vi "Send Set Room Lamp State.vi"(7 "Priority":T2=enum."Normal" caption="Message Priority (Normal)", 8 "error in (no error)":errorcluster, 9 "Value":bool, 10 "Room List":T1, 11 "Message Enqueuer in":refnum<class "Message Enqueuer.lvclass">) -> (0 "error out":errorcluster, 3 "Message Enqueuer out":refnum<class "Message Enqueuer.lvclass">)   [LabVIEW 2021, in "Light Control.lvlib" / "Set Room Lamp State Msg.lvclass"]
doc: "Sends the <b>Light Control.lvlib:Set Room Lamp State Msg.lvclass</b> message.\n\nThis message will call <b>Set Room Lamp State.vi</b> on the <b>Light Control.lvlib:Light Control.lvclass</b> actor.\n\n<b>Set Room Lamp State.vi Description</b>"
uses:
  Set Room Lamp State Msg.lvclass
  <vilib>/ActorFramework/Message Enqueuer/Message Enqueuer.lvclass
  <vilib>/ActorFramework/Message Enqueuer/Message Priority.ctl
  Light Control/Room List.ctl
  C:/Program Files (x86)/National Instruments/LabVIEW 2021/vi.lib/ActorFramework/Message/Message.lvclass
  Set Room Lamp State Msg.lvclass/Set Room Lamp State Msg.ctl
  <vilib>/ActorFramework/Message Enqueuer/Message Enqueuer.lvclass/Message Enqueuer.ctl
  <vilib>/ActorFramework/Message Priority Queue/Priority Enqueue.vi
  Light Control/Light Control.lvclass
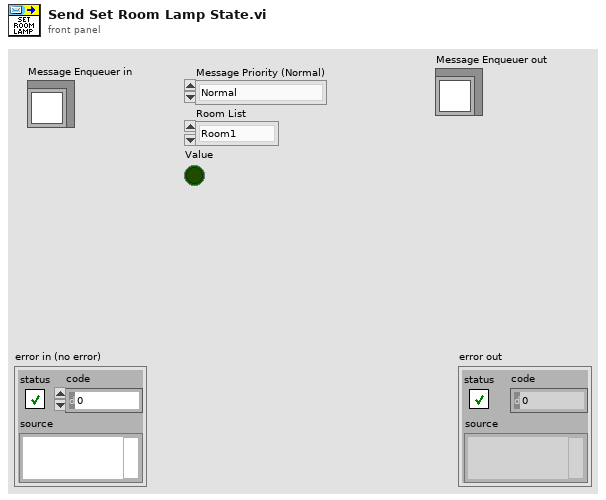
[diagram p1: front panel]
types:
  T1 = typedef "Light Control.lvlib/Light Control.lvclass/Room List.ctl" = enum16{"Room1", "Room2"}
  T2 = typedef "Actor Framework.lvlib/Message Enqueuer.lvclass/Message Priority.ctl" = enum16{"Low", "Normal", "High"}
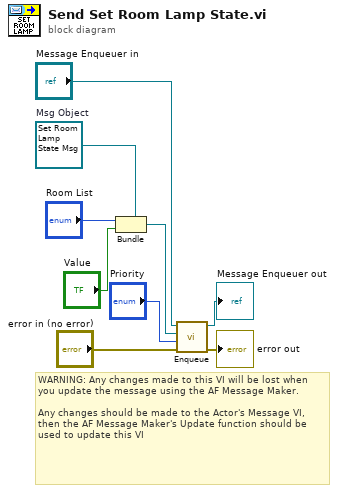
[diagram p0: block diagram]
diagram:
  w7 = refnum<class "Set Room Lamp State Msg.lvclass"> refnum  # Msg Object
  # "WARNING: Any changes made to this VI will be lost when you update the message using the AF Message Maker.\n\nAny changes should be made to the Actor's Message VI, then the AF Message Maker's Update function should be used to update this VI"
  n1 = Bundle(cluster=w7, "Room List", "Value") -> (w2:refnum<class "Set Room Lamp State Msg.lvclass">)
  n2 = call <vilib>:"Enqueue.vi"("error in (no error)"="error in (no error)", "Message Priority (Normal)"="Priority", "Message"=w2, "Message Enqueuer in"="Message Enqueuer in") -> ("error out"=→"error out":errorcluster, "Message Enqueuer out"=→"Message Enqueuer out":refnum<class "Message Enqueuer.lvclass">)  [unwired: 6 in]
